vi "Barycenter2DAuto.vi"(0 "Image":dbl[][](array[numeric]) format="%.2f") -> (1 "Bary X":dbl format="%.2f", 2 "Bary Y":dbl format="%.2f")   [LabVIEW 2009]
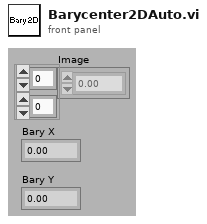
[diagram p1: front panel]
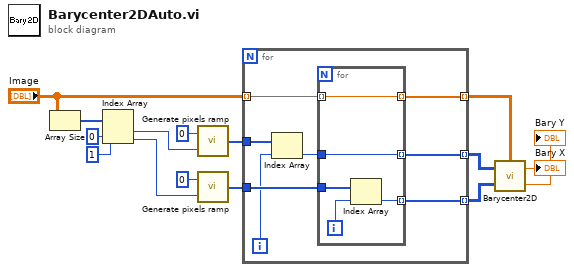
[diagram p0: block diagram]
diagram:
  n1 = Array Size(array="Image") -> (size(s)=w13:i32[])
  n2 = Index Array(array=w13, index #1=0 ("indice"), index #2=1 ("indice")) -> (element #1=w10:i32, element #2=w9:i32)
  n3 = call "Generate pixels ramp.vi"("DX"=w10, "X0"=i16 0) -> ("Ramp"=w7:i16[])
  n4 = call "Generate pixels ramp.vi"("DX"=w9, "X0"=i16 0) -> ("Ramp"=w6:i16[])
  n5 = for {
    tunnel: "Image" -> [w23] mode=indexing
    tunnel: w7 -> [w22]
    tunnel: w6 -> [w21]
    tunnel: [w18] -> w4 mode=indexing
    tunnel: [w17] -> w3 mode=indexing
    tunnel: [w16] -> w5 mode=indexing
    i -> [w20]
    n6 = Index Array(array=w22, index=w20) -> (element=w19:i16)
    n7 = for {
      tunnel: w23 -> [w24] mode=indexing
      tunnel: w21 -> [w28]
      tunnel: w19 -> [w26]
      tunnel: [w26] -> w18 mode=indexing
      tunnel: [w25] -> w17 mode=indexing
      tunnel: [w24] -> w16 mode=indexing
      i -> [w27]
      n8 = Index Array(array=w28, index=w27) -> (element=w25:i16)
    }
  }
  n9 = call "Barycenter2D.vi"("Coord Y"=w3, "Coord X"=w4, "Image"=w5) -> ("Bary Y"=→"Bary Y":dbl, "Bary X"=→"Bary X":dbl)  [unwired: 1 in]
